vi "Main.vi"(11 "Module Admin":refnum<class "Delacor_lib_QMH_Module Admin.lvclass">) -> ()   [LabVIEW 2024, in "DataViewer.lvlib"]
doc: "This template is based off of the Queued Message Handler design pattern and the Queued Message Handler project template that ships with LabVIEW.\n\nThe main difference is that the queue is private to this module and communication between modules is performed via Broadcast and Request events.\n\nRequest events are wrapped in public API methods and are handled in the Event Handling Loop (EHL) of this VI. Any module can register for Broadcast events sent by this module. The EHL generates messages based on user interface actions.\n\nThe Message Handling Loop (MHL) processes messages generated by the EHL, or by other messages. The messages are string values, so new messages can be added easily to the Message Cases case structure in the MHL. Each message cluster can also provide an optional value for Message Data, which is a variant that can be converted to whatever message-specific data is required.\n_____\nBased on DQMH Project Template 7.0.1.1316."
uses:
  DataViewer.lvlib
  <vilib>/Delacor/Delacor QMH/Libraries/Message Queue_class/Delacor_lib_QMH_Message Queue.lvclass
  Module Data--cluster.ctl
  <vilib>/Delacor/Delacor QMH/Libraries/Message Queue_class/Delacor_lib_QMH_Enqueue Message (Single).vi
  Stop Argument--cluster.ctl
  <vilib>/Delacor/Delacor QMH/Libraries/Module Admin_class/Delacor_lib_QMH_Module Admin.lvclass
  Get UI Reference (Reply Payload)--cluster.ctl
  Get UI Reference Argument--cluster.ctl
  <userlib>/_OpenG.lib/appcontrol/appcontrol.llb/openg_application_control.lvlib
  Inserted Into Subpanel Argument--cluster.ctl
  Config.ctl
  Set Config (String) Argument--cluster.ctl
  Set Config Argument--cluster.ctl
  Get config (Reply Payload)--cluster.ctl
  Get config Argument--cluster.ctl
  Get Config (String) (Reply Payload)--cluster.ctl
  Get Config (String) Argument--cluster.ctl
  Generate Dummy Data Argument--cluster.ctl
panel:
  out "Title":string
  out "Waveform Chart":dynamicdata(graph)
  out "error out":errorcluster
  out "Status":string
  in  "Simulate MHL Error":bool
  in  "Simulate EHL Error":bool
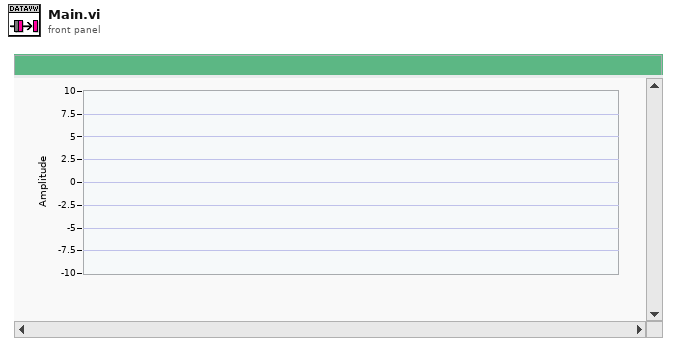
[diagram p1: front panel]
types:
  T1 = typedef "DataViewer.lvlib/Request Events--cluster.ctl" = cluster{"Stop Module":refnum<user-event>, "Show Panel":refnum<user-event>, "Hide Panel":refnum<user-event>, "Get Module Execution Status":refnum<user-event>, "Show Diagram":refnum<user-event>, "Get UI Reference":refnum<user-event>, "Inserted Into Subpanel":refnum<user-event>, "Set Config (String)":refnum<user-event>, "Set Config":refnum<user-event>, "Get config":refnum<user-event>, "Get Config (String)":refnum<user-event>, "Generate Dummy Data":refnum<user-event>}
  T2 = typedef "DataViewer.lvlib/Module Data--cluster.ctl" = cluster{"Status":string, "Config":T3}
  T3 = typedef "DataViewer.lvlib/Config.ctl" = cluster{"<ReplaceMe>":bool}
  T4 = enum32{"invalid lock state", "Not Locked", "Locked (No Password)", "Password-protected"}
  T5 = typedef "DataViewer.lvlib/Stop Argument--cluster.ctl" = cluster{"Origin":string, "Exit via Stop Module Req?":bool, "Wait for Module to stop?":bool}
  T6 = typedef "DataViewer.lvlib/Get UI Reference Argument--cluster.ctl" = cluster{"Wait Notifier":refnum<notifier>, "wait for reply":bool}
  T7 = typedef "DataViewer.lvlib/Inserted Into Subpanel Argument--cluster.ctl" = cluster{"Boolean":bool}
  T8 = typedef "DataViewer.lvlib/Set Config (String) Argument--cluster.ctl" = cluster{"XML-String":string}
  T9 = typedef "DataViewer.lvlib/Set Config Argument--cluster.ctl" = cluster{"Config":T3}
  T10 = typedef "DataViewer.lvlib/Get config Argument--cluster.ctl" = cluster{"Wait Notifier":refnum<notifier>, "wait for reply":bool}
  T11 = typedef "DataViewer.lvlib/Get Config (String) Argument--cluster.ctl" = cluster{"Wait Notifier":refnum<notifier>, "wait for reply":bool}
  T12 = typedef "DataViewer.lvlib/Generate Dummy Data Argument--cluster.ctl" = cluster{"Boolean":bool}
  T13 = enum32{"Invalid", "Standard", "Closed", "Hidden", "Minimized", "Maximized"}
  T14 = typedef "DataViewer.lvlib/Get UI Reference (Reply Payload)--cluster.ctl" = cluster{"UI VI Refnum":refnum<vi>, "error":errorcluster}
  T15 = typedef "DataViewer.lvlib/Get config (Reply Payload)--cluster.ctl" = cluster{"Config":T3, "error":errorcluster}
  T16 = typedef "DataViewer.lvlib/Get Config (String) (Reply Payload)--cluster.ctl" = cluster{"Config XML String":string, "error":errorcluster}
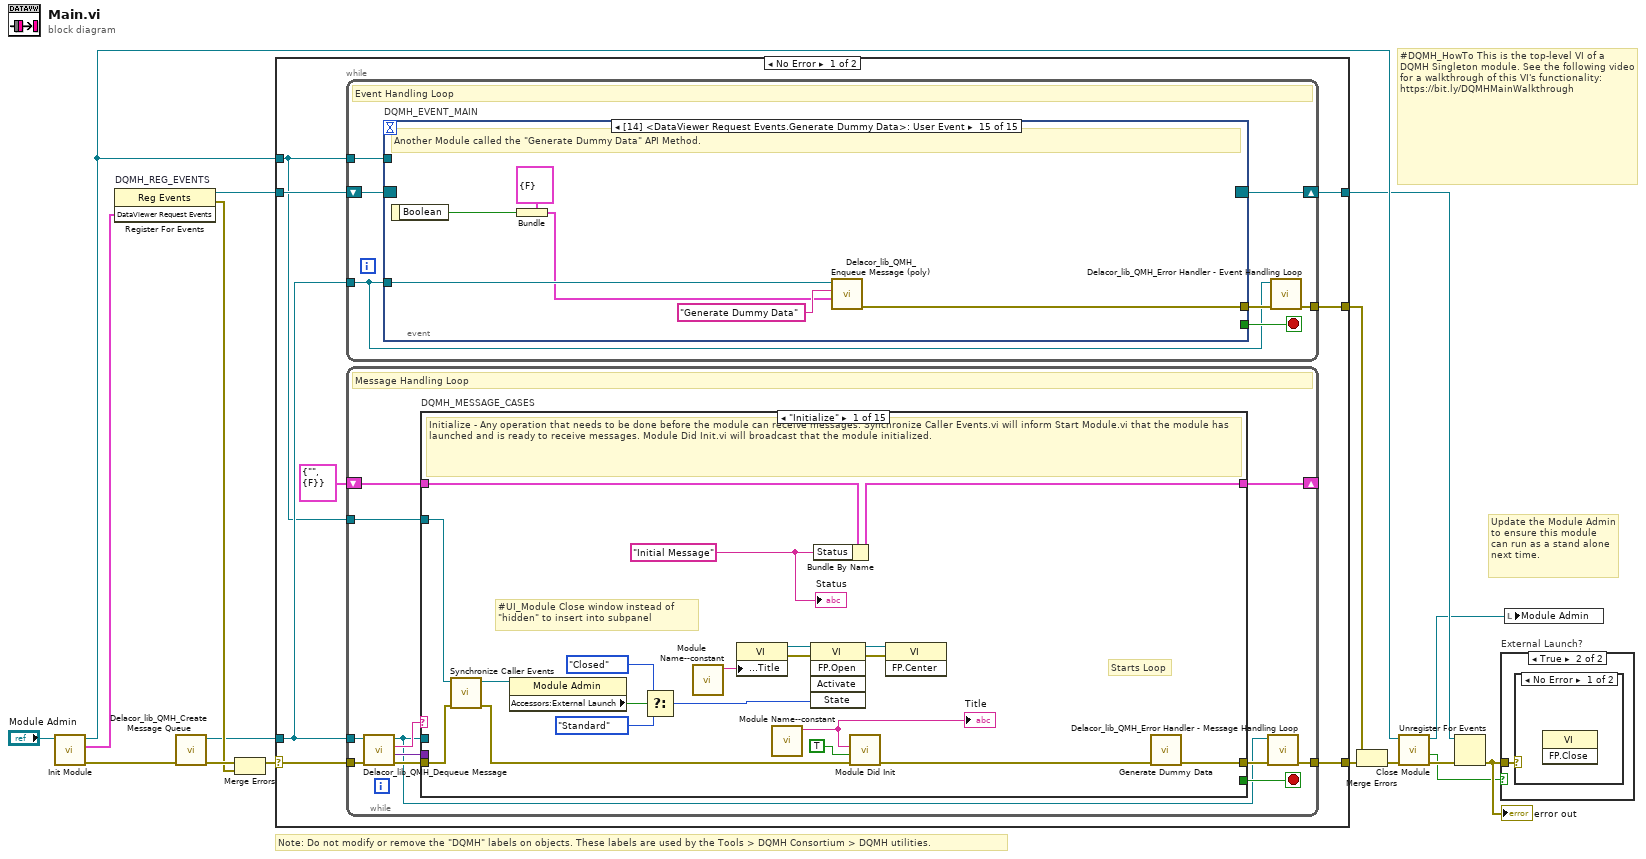
[diagram p0: block diagram]
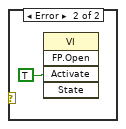
[diagram p3: hidden frame]
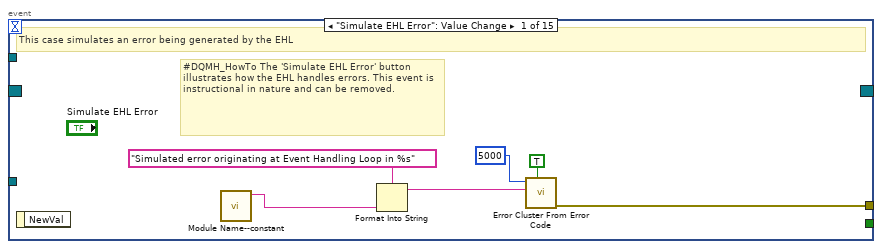
[diagram p4: hidden frame]
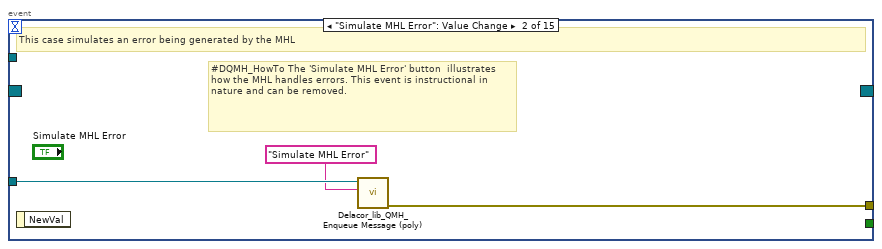
[diagram p5: hidden frame]
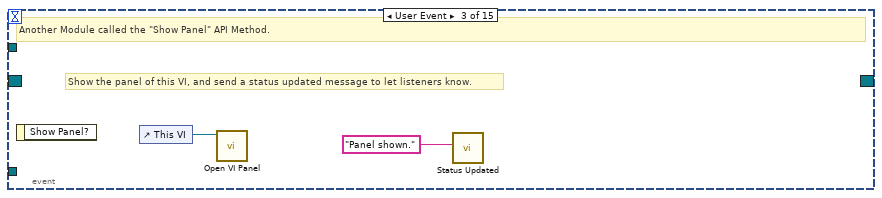
[diagram p6: hidden frame]
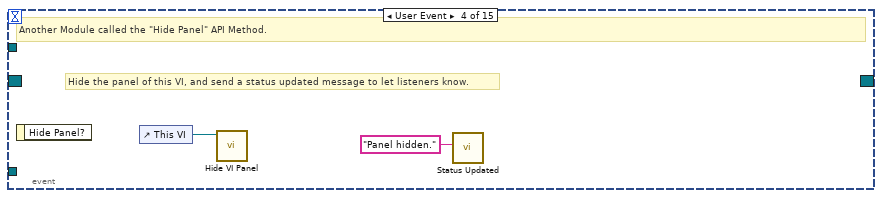
[diagram p7: hidden frame]
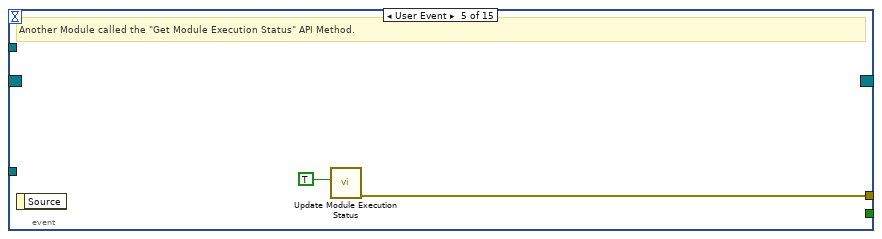
[diagram p8: hidden frame]
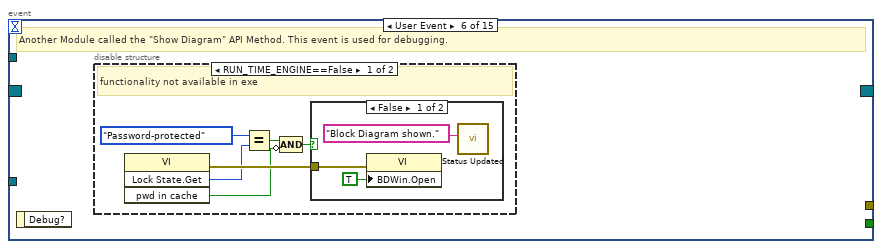
[diagram p9: hidden frame]
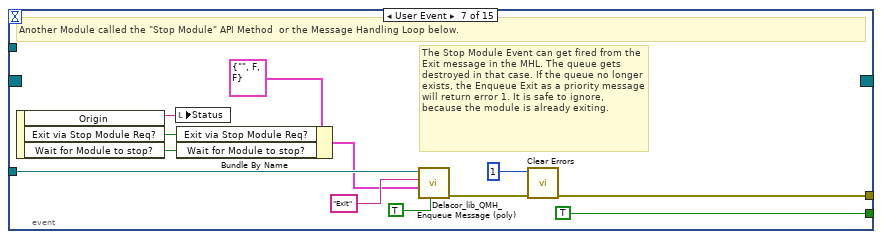
[diagram p12: hidden frame]
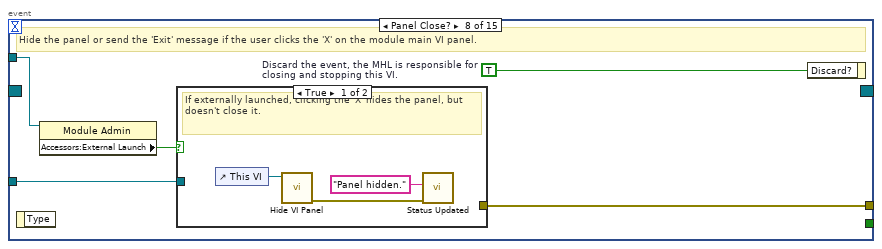
[diagram p13: hidden frame]
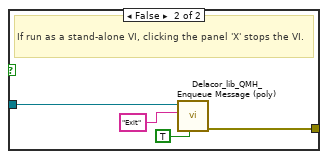
[diagram p14: hidden frame]
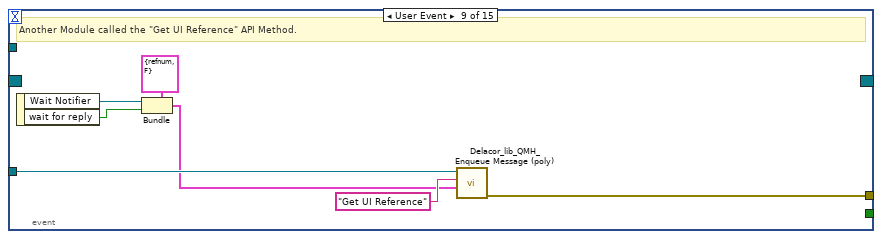
[diagram p15: hidden frame]
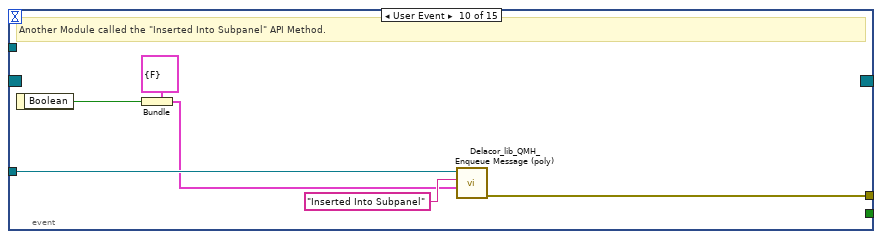
[diagram p16: hidden frame]
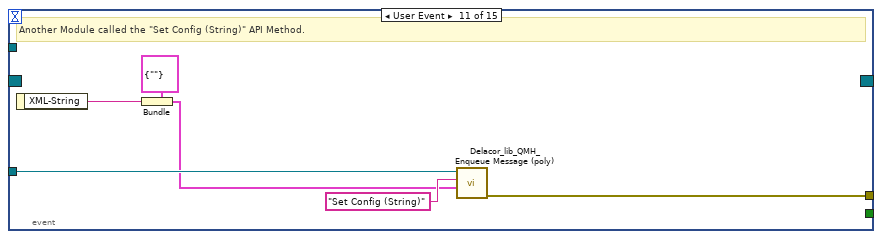
[diagram p17: hidden frame]
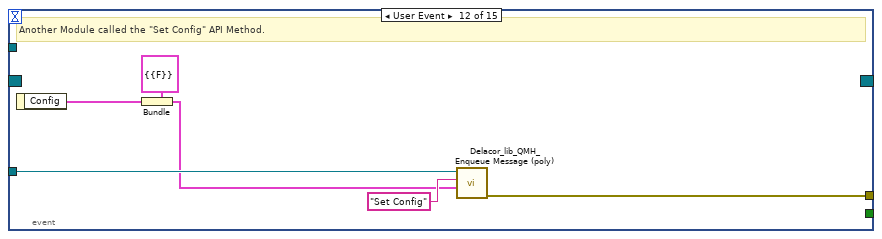
[diagram p18: hidden frame]
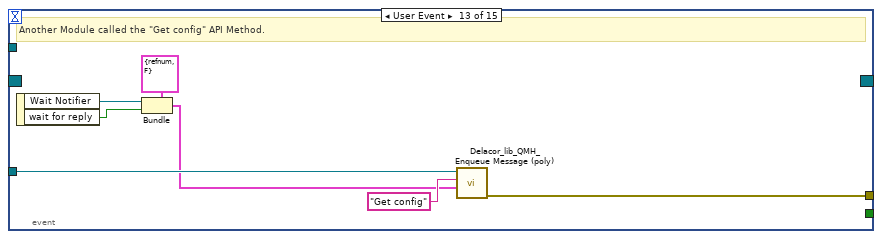
[diagram p19: hidden frame]
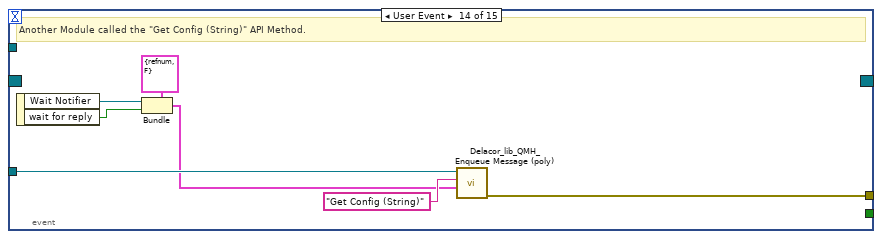
[diagram p20: hidden frame]
diagram:
  # "#DQMH_HowTo This is the top-level VI of a DQMH Singleton module. See the following video for a walkthrough of this VI's functionality: https://bit.ly/DQMHMainWalkthrough"
  # "Note: Do not modify or remove the \"DQMH\" labels on objects. These labels are used by the Tools > DQMH Consortium > DQMH utilities."
  # "Update the Module Admin to ensure this module can run as a stand alone next time."
  n1 = call "Init Module.vi"("Singleton Module Admin in"="Module Admin") -> ("error out"=w16:errorcluster, "DataViewer Request Events"=w5:T1, "Singleton Module Admin out"=w8:refnum<class "Delacor_lib_QMH_Module Admin.lvclass">)  [unwired: 8 in]
  n2 = register-events "DQMH_REG_EVENTS"(w5) -> (reference out=w6:refnum<event-registration>, error out=w9:errorcluster)  [unwired: 2 in]
  n3 = call <vilib>:"Delacor_lib_QMH_Create Message Queue.vi"("error in"=w16) -> ("error out"=w11:errorcluster, "Message Queue"=w4:refnum<class "Delacor_lib_QMH_Message Queue.lvclass">)  [unwired: 9 in]
  n4 = Merge Errors(w11, w9) -> (w10:errorcluster)
  n5 = case shown="No Error" w10 {
    selector: w10 -> [w23 w290]
    tunnel: [w25 w289] -> w17
    tunnel: [w22 w288] -> w7
    tunnel: w6 -> [w20 w288]
    tunnel: w4 -> [w19 w283]
    tunnel: [w24 _] -> w14
    tunnel: w8 -> [w18 w284]
    frame No Error {
      n6 = while {
        tunnel: w19 -> [w26]
        shift-right: [w29] -> w22
        shift-left: w20 -> [w30]
        tunnel: [w31] -> w24
        tunnel: w18 -> [w27]
        stop <- w28 stop-if-true
        # "Event Handling Loop"
        n7 = event "DQMH_EVENT_MAIN" shown="[14] <DataViewer Request Events.Generate Dummy Data>: User Event" {
          selector: w30 -> [_ _ _ _ _ _ _ _ _ _ _ _ _ _ _]
          dyn-events: [_ _ _ _ _ _ _ _ _ _ _ _ _ _ _] -> w29
          timeout: _ -> [_ _ _ _ _ _ _ _ _ _ _ _ _ _ _]
          tunnel: [_ _ _ _ _ _ TRUE ("Discard?") _ _ _ _ _ _ _ _] -> w28
          tunnel: w26 -> [_ w40 _ _ _ _ w64 w71 w87 w93 w99 w105 w112 w119 w125]
          tunnel: [w38 w41 _ _ w47 _ w67 w73 w81 w88 w94 w100 w106 w113 w120] -> w32
          tunnel: w27 -> [_ _ _ _ _ _ _ w70 _ _ _ _ _ _ _]
          event "Simulate EHL Error": Value Change {
            # "#DQMH_HowTo The 'Simulate EHL Error' button  illustrates how the EHL handles errors. This event is instructional in nature and can be removed."
            # "This case simulates an error being generated by the EHL"
            n8 = event-data() -> ()  [unwired: 1 in, 1 out]
            n9 = call "Module Name--constant.vi"() -> ("Module Name"=w35:string)  [unwired: 11 in]
            n10 = Format Into String(format string="Simulated error originating at Event Handling Loop in %s", w35) -> (resulting string=w36:string)  [unwired: 2 in, 1 out]
            n11 = call <vilib>:"Error Cluster From Error Code.vi"("show call chain? (False)"=TRUE, "error message (\"\")"=w36, "error code (0)"=5000) -> ("error out"=w38:errorcluster)  [unwired: 6 in]
          }
          event "Simulate MHL Error": Value Change {
            # "#DQMH_HowTo The 'Simulate MHL Error' button  illustrates how the MHL handles errors. This event is instructional in nature and can be removed."
            # "This case simulates an error being generated by the MHL"
            n12 = event-data() -> ()  [unwired: 1 in, 1 out]
            n13 = call-poly <vilib>:"Delacor_lib_QMH_Enqueue Message (poly).vi"("Message"="Simulate MHL Error", "Message Queue in"=w40) -> ("error out"=w41:errorcluster)  [unwired: 8 in, 1 out]
          }
          event User Event {
            # "Show the panel of this VI, and send a status updated message to let listeners know."
            # "Another Module called the \"Show Panel\" API Method."
            n14 = event-data() -> ()  [unwired: 1 in, 1 out]
            n15 = control-ref of="This VI"() -> (w43:refnum<vi>)
            n16 = call "Open VI Panel.vi"("VI"=w43) -> ()  [unwired: 10 in, 1 out]
            n17 = call "Status Updated.vi"("Status"="Panel shown." ("format string")) -> ()  [unwired: 10 in, 1 out]
          }
          event User Event {
            # "Hide the panel of this VI, and send a status updated message to let listeners know."
            # "Another Module called the \"Hide Panel\" API Method."
            n18 = event-data() -> ()  [unwired: 1 in, 1 out]
            n19 = control-ref of="This VI"() -> (w45:refnum<vi>)
            n20 = call "Hide VI Panel.vi"("VI"=w45) -> ()  [unwired: 10 in, 1 out]
            n21 = call "Status Updated.vi"("Status"="Panel hidden." ("format string")) -> ()  [unwired: 10 in, 1 out]
          }
          event User Event {
            # "Another Module called the \"Get Module Execution Status\" API Method."
            n22 = event-data() -> ()  [unwired: 1 in, 1 out]
            n23 = call "Update Module Execution Status.vi"("Running?"=TRUE) -> ("error out"=w47:errorcluster)  [unwired: 10 in]
          }
          event User Event {
            # "Another Module called the \"Show Diagram\" API Method. This event is used for debugging."
            n24 = event-data() -> ()  [unwired: 1 in, 1 out]
            n25 = disable-structure shown="RUN_TIME_ENGINE==False" {
              frame condition #0 (active) {
                # "functionality not available in exe"
                n26 = invoke on="Invoke Node" class="VI" method="Lock State.Get"() -> (error out=w53:errorcluster, "Get Lock State"=w52:T4, "pwd in cache"=w49:bool)  [unwired: 4 in, 1 out]
                n27 = Equal?(x=T4."Password-protected", y=w52) -> (x = y?=w50:bool)
                n28 = Compound Arithmetic op=AND(w50, invert w49) -> (w48:bool)
                n29 = case shown="False" w48 {
                  tunnel: w53 -> [w56 _]
                  frame False {
                    n30 = property on="Property Node" class="VI"(error in=w56, "BDWin.Open"=TRUE ("Block Diagram Window:Open")) -> ()  [unwired: 1 in, 2 out]
                    n31 = call "Status Updated.vi"("Status"="Block Diagram shown." ("format string")) -> ()  [unwired: 10 in, 1 out]
                  }
                  frame True {
                    # "Password-protected VI, and the password is not in the cache. Do not show the diagram."
                  }
                }
              }
              frame condition #1 {
              }
            }
          }
          event User Event {
            # "The Stop Module Event can get fired from the Exit message in the MHL. The queue gets destroyed in that case. If the queue no longer exists, the Enqueue Exit as a priority message will return error 1. It is safe to ignore, because the module is already exiting."
            # "Another Module called the \"Stop Module\" API Method  or the Message Handling Loop below."
            n32 = event-data() -> ("Origin"=w63:string, "Exit via Stop Module Req?"=w59:bool, "Wait for Module to stop?"=w58:bool)  [unwired: 1 in]
            n33 = local write "Status"(w63) -> ()
            n34 = Bundle By Name(cluster=T5 {"Origin"="", "Exit via Stop Module Req?"=FALSE, "Wait for Module to stop?"=FALSE} ("Stop Argument"), "Exit via Stop Module Req?"=w59, "Wait for Module to stop?"=w58) -> (w57:T5)
            n35 = call-poly <vilib>:"Delacor_lib_QMH_Enqueue Message (poly).vi"("Priority Message? (F)"=TRUE, "Message Data"=w57, "Message"="Exit", "Message Queue in"=w64) -> ("error out"=w68:errorcluster)  [unwired: 6 in, 1 out]
            n36 = call <vilib>:"Clear Errors.vi"("error in (no error)"=w68, "specific error code to clear (0: all)"=1) -> ("error out"=w67:errorcluster)  [unwired: 4 in, 1 out]
          }
          event Panel Close? {
            w72 = TRUE  # Discard the event, the MHL is responsible for closing and stopping this VI.
            # "Hide the panel or send the 'Exit' message if the user clicks the 'X' on the module main VI panel."
            n37 = event-data() -> ()  [unwired: 1 in, 1 out]
            n38 = property on="Property Node" class="Module Admin"(reference=w70) -> ("Accessors:External Launch"=w69:bool)  [unwired: 1 in, 2 out]
            n39 = case shown="True" w69 {
              tunnel: w71 -> [_ w79]
              tunnel: [_ w80] -> w73
              frame True {
                # "If externally launched, clicking the 'X' hides the panel, but doesn't close it."
                n40 = control-ref of="This VI"() -> (w76:refnum<vi>)
                n41 = call "Hide VI Panel.vi"("VI"=w76) -> ("error out"=w74:errorcluster)  [unwired: 10 in]
                n42 = call "Status Updated.vi"("error in"=w74, "Status"="Panel hidden." ("format string")) -> ()  [unwired: 9 in, 1 out]
              }
              frame False {
                # "If run as a stand-alone VI, clicking the panel 'X' stops the VI."
                n43 = call-poly <vilib>:"Delacor_lib_QMH_Enqueue Message (poly).vi"("Priority Message? (F)"=TRUE, "Message"="Exit", "Message Queue in"=w79) -> ("error out"=w80:errorcluster)  [unwired: 7 in, 1 out]
              }
            }
            n44 = event-data ("Event Filter Node")("Discard?"=w72) -> ()  [unwired: 1 in, 1 out]
          }
          event User Event {
            # "Another Module called the \"Get UI Reference\" API Method."
            n45 = event-data() -> ("Wait Notifier"=w83:refnum<notifier>, "wait for reply"=w82:bool)  [unwired: 1 in]
            n46 = Bundle(cluster=T6 {"Wait Notifier"=refnum, "wait for reply"=FALSE} ("Get UI Reference Argument"), "Wait Notifier"=w83, "wait for reply"=w82) -> (w84:T6)
            n47 = call-poly <vilib>:"Delacor_lib_QMH_Enqueue Message (poly).vi"("Message Data"=w84, "Message"="Get UI Reference", "Message Queue in"=w87) -> ("error out"=w81:errorcluster)  [unwired: 7 in, 1 out]
          }
          event User Event {
            # "Another Module called the \"Inserted Into Subpanel\" API Method."
            n48 = event-data() -> ("Boolean"=w89:bool)  [unwired: 1 in]
            n49 = Bundle(cluster=T7 {"Boolean"=FALSE} ("Inserted Into Subpanel Argument"), "Boolean"=w89) -> (w90:T7)
            n50 = call-poly <vilib>:"Delacor_lib_QMH_Enqueue Message (poly).vi"("Message Data"=w90, "Message"="Inserted Into Subpanel", "Message Queue in"=w93) -> ("error out"=w88:errorcluster)  [unwired: 7 in, 1 out]
          }
          event User Event {
            # "Another Module called the \"Set Config (String)\" API Method."
            n51 = event-data() -> ("XML-String"=w95:string)  [unwired: 1 in]
            n52 = Bundle(cluster=T8 {"XML-String"=""} ("Set Config (String) Argument"), "XML-String"=w95) -> (w96:T8)
            n53 = call-poly <vilib>:"Delacor_lib_QMH_Enqueue Message (poly).vi"("Message Data"=w96, "Message"="Set Config (String)", "Message Queue in"=w99) -> ("error out"=w94:errorcluster)  [unwired: 7 in, 1 out]
          }
          event User Event {
            # "Another Module called the \"Set Config\" API Method."
            n54 = event-data() -> ("Config"=w101:T3)  [unwired: 1 in]
            n55 = Bundle(cluster=T9 {"Config"={"<ReplaceMe>"=FALSE}} ("Set Config Argument"), "Config"=w101) -> (w102:T9)
            n56 = call-poly <vilib>:"Delacor_lib_QMH_Enqueue Message (poly).vi"("Message Data"=w102, "Message"="Set Config", "Message Queue in"=w105) -> ("error out"=w100:errorcluster)  [unwired: 7 in, 1 out]
          }
          event User Event {
            # "Another Module called the \"Get config\" API Method."
            n57 = event-data() -> ("Wait Notifier"=w108:refnum<notifier>, "wait for reply"=w107:bool)  [unwired: 1 in]
            n58 = Bundle(cluster=T10 {"Wait Notifier"=refnum, "wait for reply"=FALSE} ("Get config Argument"), "Wait Notifier"=w108, "wait for reply"=w107) -> (w109:T10)
            n59 = call-poly <vilib>:"Delacor_lib_QMH_Enqueue Message (poly).vi"("Message Data"=w109, "Message"="Get config", "Message Queue in"=w112) -> ("error out"=w106:errorcluster)  [unwired: 7 in, 1 out]
          }
          event User Event {
            # "Another Module called the \"Get Config (String)\" API Method."
            n60 = event-data() -> ("Wait Notifier"=w115:refnum<notifier>, "wait for reply"=w114:bool)  [unwired: 1 in]
            n61 = Bundle(cluster=T11 {"Wait Notifier"=refnum, "wait for reply"=FALSE} ("Get Config (String) Argument"), "Wait Notifier"=w115, "wait for reply"=w114) -> (w116:T11)
            n62 = call-poly <vilib>:"Delacor_lib_QMH_Enqueue Message (poly).vi"("Message Data"=w116, "Message"="Get Config (String)", "Message Queue in"=w119) -> ("error out"=w113:errorcluster)  [unwired: 7 in, 1 out]
          }
          event User Event {
            # "Another Module called the \"Generate Dummy Data\" API Method."
            n63 = event-data() -> ("Boolean"=w121:bool)  [unwired: 1 in]
            n64 = Bundle(cluster=T12 {"Boolean"=FALSE} ("Generate Dummy Data Argument"), "Boolean"=w121) -> (w122:T12)
            n65 = call-poly <vilib>:"Delacor_lib_QMH_Enqueue Message (poly).vi"("Message Data"=w122, "Message"="Generate Dummy Data", "Message Queue in"=w125) -> ("error out"=w120:errorcluster)  [unwired: 7 in, 1 out]
          }
        }
        n66 = call-dynamic "Delacor_lib_QMH_Error Handler - Event Handling Loop.vi"("error in"=w32, "Message Queue in"=w26) -> ("dup error in"=w31:errorcluster)  [unwired: 8 in, 1 out]
      }
      n67 = while {
        tunnel: w19 -> [w126]
        shift-right: [w134] -> _
        shift-left: T2 {"Status"="", "Config"={"<ReplaceMe>"=FALSE}} ("Data Cluster") -> [w135]
        tunnel: w23 -> [w137]
        tunnel: [w129] -> w25
        tunnel: w18 -> [w130]
        stop <- w133 stop-if-true
        # "Message Handling Loop"
        n68 = call-dynamic "Delacor_lib_QMH_Dequeue Message.vi"("error in"=w137, "Message Queue in"=w126) -> ("error out"=w136:errorcluster, "Message Data"=w131:variant, "Message"=w132:string, "Message Queue out"=w127:refnum<class "Delacor_lib_QMH_Message Queue.lvclass">)  [unwired: 6 in]
        n69 = case "DQMH_MESSAGE_CASES" shown="\"Initialize\"" w132 {
          selector: w132 -> [_ _ _ _ _ _ _ _ _ _ _ _ _ _ w278]
          tunnel: w127 -> [_ _ _ _ _ _ _ _ _ _ _ _ w244 w266 _]
          tunnel: w136 -> [w155 w159 w171 w174 w186 w192 w204 w219 w225 w229 w231 w240 w251 w272 w281]
          tunnel: [w138 w159 w161 w174 w180 w190 w195 w210 w224 w228 w231 w239 w247 w267 w282] -> w128
          tunnel: w135 -> [w145 w158 w170 w175 w185 w191 w194 w209 w226 w227 w230 w237 w246 w265 w279]
          tunnel: [w144 w158 w170 w175 w177 w191 w194 w209 w226 w227 w230 w237 w246 w265 w279] -> w134
          tunnel: [_ _ _ _ _ _ _ _ _ _ _ _ _ w264 _] -> w133
          tunnel: w131 -> [_ _ w168 _ w183 w189 w202 w217 _ _ _ _ w245 w263 _]
          tunnel: w130 -> [w146 _ _ _ _ _ _ _ _ _ _ _ w243 w258 _]
          frame "Initialize" {
            w141 = "Initial Message" ("Initial Message")
            # "Starts Loop"
            # "#UI_Module Close window instead of\n\"hidden\" to insert into subpanel"
            # "Initialize - Any operation that needs to be done before the module can receive messages. Synchronize Caller Events.vi will inform Start Module.vi that the module has launched and is ready to receive messages. Module Did Init.vi will broadcast that the module initialized."
            n70 = call "Synchronize Caller Events.vi"("error in"=w155, "Singleton Module Admin in"=w146) -> ("error out"=w154:errorcluster, "Singleton Module Admin out"=w142:refnum<class "Delacor_lib_QMH_Module Admin.lvclass">)  [unwired: 8 in]
            n71 = property on="Property Node" class="Module Admin"(reference=w142) -> ("Accessors:External Launch"=w150:bool)  [unwired: 1 in, 2 out]
            n72 = Select(t=T13."Closed" ("State"), s=w150, f=T13."Standard" ("State")) -> (s? t:f=w147:T13)
            n73 = call "Module Name--constant.vi"() -> ("Module Name"=w153:string)  [unwired: 11 in]
            n74 = property on="Property Node" class="VI"("Front Panel.Title"=w153) -> (reference out=w152:refnum<vi>, error out=w157:errorcluster)  [unwired: 2 in]
            n75 = call "Module Name--constant.vi"() -> ("Module Name"=w140:string)  [unwired: 11 in]
            "Title" <- w140
            n76 = invoke on="Invoke Node" class="VI" method="FP.Open"(reference=w152, error in=w157, "State"=w147) -> (reference out=w151:refnum<vi>, error out=w156:errorcluster)  [unwired: 2 in, 3 out]
            n77 = Bundle By Name(cluster=w145, "Status"=w141) -> (w144:T2)
            n78 = call "Module Did Init.vi"("error in"=w154, "Initialized?"=TRUE, "Origin"=w140) -> ("error out"=w139:errorcluster)  [unwired: 8 in]
            n79 = invoke on="Invoke Node" class="VI" method="FP.Center"(reference=w151, error in=w156) -> ()  [unwired: 1 in, 3 out]
            n80 = call "Generate Dummy Data.vi"("error in"=w139) -> ("error out"=w138:errorcluster)  [unwired: 10 in]
            "Status" <- w141
          }
          frame "---Module Specific---" {
            # "Separator -- The following cases handle messages specific to this Module."
          }
          frame "Get UI Reference" {
            # "Returns the VI Reference of the UI of the Module, usually the main.vi. Use this to insert the Module into a sub-panel."
            n81 = Variant To Data(error in=w171, type=T6 {"Wait Notifier"=refnum, "wait for reply"=FALSE} ("Get UI Reference Argument"), Variant=w168) -> (data=w166:T6, error out=w169:errorcluster)
            n82 = Unbundle By Name(w166) -> ("Wait Notifier"=w165:refnum<notifier>, "wait for reply"=w164:bool)
            n83 = call <userlib>:"Current VIs Reference__ogtk.vi"() -> ("Current VI's reference"=w160:refnum<vi>)  [unwired: 5 in]
            n84 = Bundle By Name(cluster=T14 {"UI VI Refnum"=refnum, "error"={"status"=FALSE, "code"=0, "source"=""}} ("Get UI Reference (Reply Payload)"), "UI VI Refnum"=w160) -> (w163:T14)
            n85 = Merge Errors(w169) -> (w161:errorcluster)
            n86 = case "DQMH_FIRE_NOTIFIER" shown="True" w164 {
              tunnel: w165 -> [_ w173]
              tunnel: w163 -> [_ w172]
              frame False {
              }
              frame True {
                n87 = Send Notification(notification=w172, notifier=w173) -> ()  [unwired: 1 in, 2 out]
              }
            }
          }
          frame "Inserted Into Subpanel" {
            # "#UI_Module Update UI when inserted into a subpanel"
            # "This Request is called when the UI VI is inserted into a subpanel."
          }
          frame "Set Config (String)" {
            # "Sets the config data by String of the flattened config.ctl cluster."
            n88 = Variant To Data(error in=w186, type=T8 {"XML-String"=""} ("Set Config (String) Argument"), Variant=w183) -> (data=w181:T8, error out=w184:errorcluster)
            n89 = Unbundle By Name(w181) -> ("XML-String"=w179:string)
            n90 = Unflatten From XML(xml string=w179, type=T3 {"<ReplaceMe>"=FALSE} ("Config"), error in (no error)=w184) -> (value=w176:T3, error out=w180:errorcluster)
            n91 = Bundle By Name(cluster=w185, "Config"=w176) -> (w177:T2)
          }
          frame "Set Config" {
            # "#CodeNeeded\n1. Configure this Message Case for handling the \"Set Config\" message.\n2. Delete or edit this label when done."
            # "Sets the config data for the module."
            n92 = Variant To Data(error in=w192, type=T9 {"Config"={"<ReplaceMe>"=FALSE}} ("Set Config Argument"), Variant=w189) -> (data=w187:T9, error out=w190:errorcluster)
            n93 = Unbundle By Name(w187) -> ()  [unwired: 1 out]
          }
          frame "Get config" {
            # "Returns the modules Config."
            n94 = Variant To Data(error in=w204, type=T10 {"Wait Notifier"=refnum, "wait for reply"=FALSE} ("Get config Argument"), Variant=w202) -> (data=w200:T10, error out=w203:errorcluster)
            n95 = Unbundle By Name(w200) -> ("Wait Notifier"=w199:refnum<notifier>, "wait for reply"=w198:bool)
            n96 = Unbundle By Name(w194) -> ("Config"=w193:T3)
            n97 = Bundle By Name(cluster=T15 {"Config"={"<ReplaceMe>"=FALSE}, "error"={"status"=FALSE, "code"=0, "source"=""}} ("Get config (Reply Payload)"), "Config"=w193) -> (w197:T15)
            n98 = Merge Errors(w203) -> (w195:errorcluster)
            n99 = case "DQMH_FIRE_NOTIFIER" shown="True" w198 {
              tunnel: w199 -> [_ w206]
              tunnel: w197 -> [_ w205]
              frame False {
              }
              frame True {
                n100 = Send Notification(notification=w205, notifier=w206) -> ()  [unwired: 1 in, 2 out]
              }
            }
          }
          frame "Get Config (String)" {
            # "Returns the modules config as an xml string."
            n101 = Variant To Data(error in=w219, type=T11 {"Wait Notifier"=refnum, "wait for reply"=FALSE} ("Get Config (String) Argument"), Variant=w217) -> (data=w215:T11, error out=w218:errorcluster)
            n102 = Unbundle By Name(w215) -> ("Wait Notifier"=w214:refnum<notifier>, "wait for reply"=w213:bool)
            n103 = Unbundle By Name(w209) -> ("Config"=w208:T3)
            n104 = Flatten To XML(6:w208) -> (2:w207:string)
            n105 = Bundle By Name(cluster=T16 {"Config XML String"="", "error"={"status"=FALSE, "code"=0, "source"=""}} ("Get Config (String) (Reply Payload)"), "Config XML String"=w207) -> (w212:T16)
            n106 = Merge Errors(w218) -> (w210:errorcluster)
            n107 = case "DQMH_FIRE_NOTIFIER" shown="True" w213 {
              tunnel: w214 -> [_ w221]
              tunnel: w212 -> [_ w220]
              frame False {
              }
              frame True {
                n108 = Send Notification(notification=w220, notifier=w221) -> ()  [unwired: 1 in, 2 out]
              }
            }
          }
          frame "Generate Dummy Data" {
            # "Generates dummy data on the plot"
            n109 = Wait (ms)(milliseconds to wait=u32 100) -> ()  [unwired: 1 out]
            n110 = call "Simulate Signal"() -> ("Sine"=→"Waveform Chart":dynamicdata)  [unwired: 14 in, 1 out]
            n111 = call "Generate Dummy Data.vi"("error in"=w225) -> ("error out"=w224:errorcluster)  [unwired: 10 in]
          }
          frame "---Copy This Frame---" {
            # "Duplicate this frame when creating new messages.  Change this comment in the duplicated frame to describe this message."
            n112 = Merge Errors(w229) -> (w228:errorcluster)
          }
          frame "---Exit and Error Handling---" {
            # "Separator - The following cases handle errors and exit messages."
          }
          frame "Simulate MHL Error" {
            # "#DQMH_HowTo The 'Simulate MHL Error' button  illustrates how the MHL handles errors. This event is instructional in nature and can be removed."
            # "Simulate an error occurring at the MHL"
            n113 = call "Module Name--constant.vi"() -> ("Module Name"=w233:string)  [unwired: 11 in]
            n114 = Format Into String(format string="Simulated error originating at Message Handling Loop in %s", w233) -> (resulting string=w234:string)  [unwired: 2 in, 1 out]
            n115 = call <vilib>:"Error Cluster From Error Code.vi"("show call chain? (False)"=TRUE, "error message (\"\")"=w234, "error code (0)"=5001) -> ("error out"=w238:errorcluster)  [unwired: 6 in]
            n116 = Merge Errors(w240, w238) -> (w239:errorcluster)
          }
          frame "Error" {
            # "Error - Check the error message data and respond accordingly. This message is sent by the \"Error Handler\" VIs at the end of each loop in this application."
            n117 = property on="Property Node" class="Module Admin"(reference=w243) -> ("Accessors:External Launch"=w242:bool)  [unwired: 1 in, 2 out]
            n118 = Variant To Data(error in=w251, type=errorcluster {"status"=FALSE, "code"=0, "source"=""} ("error constant"), Variant=w245) -> (data=w241:errorcluster, error out=w249:errorcluster)
            n119 = local write "error out"(w241) -> ()
            n120 = call "Error Reported.vi"("Error"=w241) -> ()  [unwired: 10 in, 1 out]
            n121 = case shown="False" w242 {
              tunnel: [w256 _] -> w248
              tunnel: w244 -> [w254 _]
              tunnel: w241 -> [w255 _]
              frame False {
                n122 = disable-structure shown="Default" {
                  disable-tunnel: w255 -> [w257 _]
                  frame condition #0 (active) {
                    # "If the module is running standalone, then pop up an error dialog and call the \"Exit\" message."
                    n123 = call <vilib>:"Simple Error Handler.vi"("error in (no error)"=w257) -> ()  [unwired: 4 in, 5 out]
                  }
                  frame condition #1 {
                    # "To prevent the Simple Error Handler VI from being loaded (e.g. when deploying to a Real-Time target), add the Conditional Disable Symbol \"DQMH_Disable_SEH\" to your project and set it to TRUE."
                  }
                }
                n124 = call-poly <vilib>:"Delacor_lib_QMH_Enqueue Message (poly).vi"("Priority Message? (F)"=TRUE, "Message"="Exit", "Message Queue in"=w254) -> ("error out"=w256:errorcluster)  [unwired: 7 in, 1 out]
              }
              frame True {
                # "If the module was launched externally, calling the Error Reported broadcast VI is the only action performed by the \"Error\" message. The module's caller can then process the error appropriately."
              }
            }
            n125 = Merge Errors(w249, w248) -> (w247:errorcluster)
          }
          frame "Exit" {
            w262 = 91  # 91: not all Exit messages will have an argument
            w264 = TRUE  # Stop the VI
            # "Release the message queue reference"
            # "Exit - Exit the application."
            n126 = Variant To Data(error in=w272, type=T5 {"Origin"="", "Exit via Stop Module Req?"=FALSE, "Wait for Module to stop?"=FALSE} ("Stop Argument"), Variant=w263) -> (data=w260:T5, error out=w269:errorcluster)
            n127 = call <vilib>:"Clear Errors.vi"("error in (no error)"=w269, "specific error code to clear (0: all)"=w262) -> ("error out"=w271:errorcluster)  [unwired: 4 in, 1 out]
            n128 = control-ref of="This VI"() -> (w259:refnum<vi>)
            n129 = call-dynamic "Delacor_lib_QMH_Release Message Queue.vi"("error in"=w271, "Message Queue"=w266) -> ("error out"=w270:errorcluster)  [unwired: 9 in]
            n130 = call "Handle Exit.vi"("Stop Argument"=w260, "Admin in"=w258, "VI reference"=w259) -> ("error out"=w268:errorcluster)  [unwired: 7 in, 1 out]
            n131 = Merge Errors(w270, w268) -> (w267:errorcluster)
            n132 = call "Error Reported.vi"("Error"=w267) -> ()  [unwired: 10 in, 1 out]
          }
          frame Default {
            # "'Default' case only runs if there is a message that isn't defined in any of the other cases.  Output a programming error."
            n133 = call "Module Name--constant.vi"() -> ("Module Name"=w277:string)  [unwired: 11 in]
            n134 = Format Into String(format string="The invalid message string \"%s\" was received in the Message Handling Loop for module \"%s\".", w278, w277) -> (resulting string=w273:string)  [unwired: 2 in, 1 out]
            n135 = call <vilib>:"Error Cluster From Error Code.vi"("show call chain? (False)"=TRUE, "error message (\"\")"=w273, "error code (0)"=1) -> ("error out"=w280:errorcluster)  [unwired: 6 in]
            n136 = Merge Errors(w281, w280) -> (w282:errorcluster)
          }
        }
        n137 = call-dynamic "Delacor_lib_QMH_Error Handler - Message Handling Loop.vi"("error in"=w128, "Message Queue in"=w127) -> ("dup error in"=w129:errorcluster)  [unwired: 8 in, 1 out]
      }
    }
    frame Error {
      # "Synchronize Caller Events.vi will inform Start Module.vi that the module has launched and will let the code calling Start Module.vi register for broadcasts and would permit the caller receive the broadcast that an error occurred at launch time."
      n138 = call-dynamic "Delacor_lib_QMH_Release Message Queue.vi"("error in"=w290, "Message Queue"=w283) -> ("error out"=w289:errorcluster)  [unwired: 9 in]
      n139 = call "Synchronize Caller Events.vi"("Singleton Module Admin in"=w284) -> ("error out"=w291:errorcluster)  [unwired: 9 in, 1 out]
      n140 = call "Module Name--constant.vi"() -> ("Module Name"=w287:string)  [unwired: 11 in]
      n141 = Format Into String(format string="An error occurred during initialization. %s is no longer running.", w287) -> (resulting string=w285:string)  [unwired: 2 in, 1 out]
      n142 = Merge Errors(w289, w291) -> (w292:errorcluster)
      n143 = call "Error Reported.vi"("Additional Information"=w285, "Error"=w292) -> ()  [unwired: 9 in, 1 out]
    }
  }
  n144 = Merge Errors(w14, w17) -> (w13:errorcluster)
  n145 = call "Close Module.vi"("error in"=w13, "Module Admin in"=w8) -> ("error out"=w15:errorcluster, "External Launch"=w1:bool, "Module Admin out"=w2:refnum<class "Delacor_lib_QMH_Module Admin.lvclass">)  [unwired: 7 in]
  n146 = Unregister For Events(event registration refnum=w7, error in=w15) -> (error out=w12:errorcluster)
  "error out" <- w12
  n147 = case "External Launch?" shown="True" w1 {
    tunnel: w12 -> [_ w293]
    frame False {
    }
    frame True {
      n148 = case shown="No Error" w293 {
        frame No Error {
          n149 = invoke on="Invoke Node" class="VI" method="FP.Close"() -> ()  [unwired: 3 in, 3 out]
        }
        frame Error {
          n150 = invoke on="Invoke Node" class="VI" method="FP.Open"("Activate"=TRUE ("Activate?")) -> ()  [unwired: 4 in, 5 out]
        }
      }
    }
  }
  n151 = local write "Module Admin"(w2) -> ()
